vi "XYGraph.vi"(8 "Last official draw":i64[](array[numeric]), 9 "stop":bool, 10 "Row":i64) -> (0 "This row":i64[](array[numeric]), 2 "Appended array":cluster{i32[], "Last official draw":i64[]}[](array[cluster]), 3 "Draw Num":i32, 11 "Java file":i64[][](array[numeric]))   [LabVIEW 2023]
panel:
  out "output cluster":cluster{i32[], "Java file":i64[]}
  in  "Yor Suppose":i64[](array[numeric])
  out "XY Graph 3":cluster{i32[], "Last official draw":i64[]}[](graph)
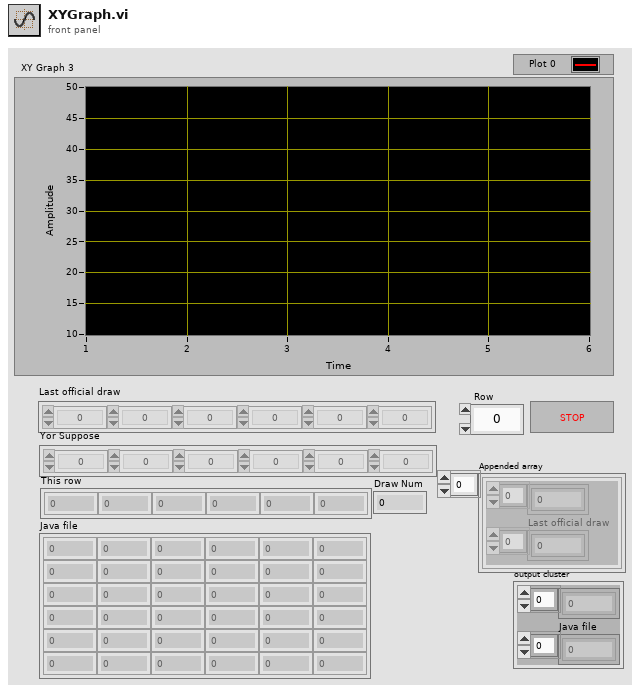
[diagram p1: front panel]
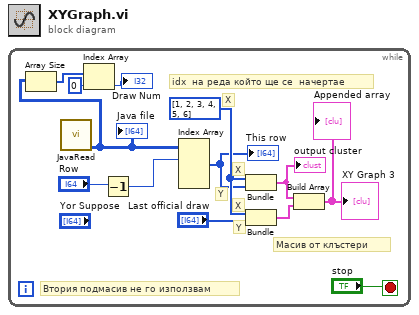
[diagram p0: block diagram]
diagram:
  n1 = while {
    stop <- "stop" stop-if-true
    w6 = i32[] [1, 2, 3, 4, 5, 6]
    # "X"
    # "X"
    # "Y"
    # "Y"
    # "X"
    # "Масив от клъстери"
    # "Втория подмасив не го използвам"
    # "idx  на реда който ще се  начертае"
    n2 = call "JavaRead.vi"() -> ("Java file"=w4:i64[][])  [unwired: 10 in, 1 out]
    "Java file" <- w4
    n3 = Array Size(array=w4) -> (size(s)=w3:i32[])
    n4 = Index Array(array=w3, index=0) -> (element=→"Draw Num":i32)
    n5 = Decrement(x="Row") -> (x-1=w11:i64)
    n6 = Index Array "Index Array"(array=w4, index (row) #1=w11) -> (element #1=w5:i64[])  [unwired: 3 in, 1 out]
    "This row" <- w5
    n7 = Bundle(w6, "Java file"=w5) -> (w9:cluster{i32[], "Java file":i64[]})  [unwired: 1 in]
    "output cluster" <- w9
    n8 = Bundle(w6, "Last official draw"="Last official draw") -> (w8:cluster{i32[], "Last official draw":i64[]})  [unwired: 1 in]
    n9 = Build Array(w9, w8) -> (→"XY Graph 3" →"Appended array":cluster{i32[], "Last official draw":i64[]}[])
  }
